vi "VISAGlobal.vi"() -> ()   [LabVIEW 2018]
panel:
  in  "VISA":refnum<visa-resource-name>
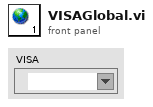
[diagram p1: front panel]
diagram:
